vi "Pixmap Probe.vi"(1 "image data":T1) -> (0 "Pause if TRUE":bool)   [LabVIEW 2020]
doc: "Displays the picture and includes information about the width, height, and image color depth of the input picture."
uses:
  <vilib>/picture/picture.llb/imagedata.ctl
panel:
  in  "format string":string="%d bits"
  in  "Tab Control":enum32{"Image   ", "Properties     "}(tab)
  out "Picture":picture
  in  "system palette":string="No color table information included. Default system palette will be used."
  out "Two color table":u32[](array[colorbox])
  out "16.4 million colors":picture
  out "Image Color Depth:":string
  out "256 color table":u32[][](array[colorbox])
  out "Height:":i16
  out "Width:":i16
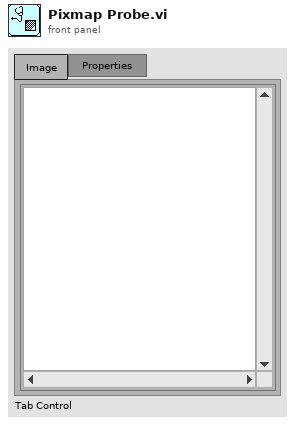
[diagram p1: front panel]
types:
  T1 = typedef "imagedata.ctl" = cluster{"image type":i32, "image depth":i32, "image":u8[], "mask":u8[], "colors":u32[], "Rectangle":cluster{"left":i16, "top":i16, "right":i16, "bottom":i16}}
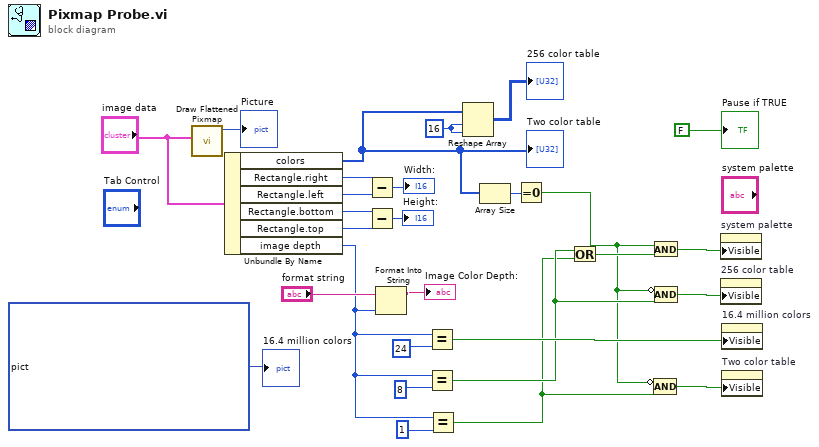
[diagram p0: block diagram]
diagram:
  w3 = 16 ("dimension size")
  n1 = call <vilib>:"Draw Flattened Pixmap.vi"("image data"="image data") -> ("new picture"=→"Picture":picture)  [unwired: 8 in]
  n2 = Unbundle By Name("image data") -> ("colors"=w9:u32[], "Rectangle.right"=w27:i16, "Rectangle.left"=w26:i16, "Rectangle.bottom"=w24:i16, "Rectangle.top"=w23:i16, "image depth"=w10:i32)
  "Two color table" <- w9
  n3 = Subtract(x=w27, y=w26) -> (x-y=→"Width:":i16)
  n4 = Subtract(x=w24, y=w23) -> (x-y=→"Height:":i16)
  n5 = Format Into String(format string="format string", w10) -> (resulting string=→"Image Color Depth:":string)  [unwired: 2 in, 1 out]
  n6 = Equal?(x=w10, y=u8 24) -> (x = y?=w12:bool)
  n7 = Equal?(x=w10, y=u8 8) -> (x = y?=w6:bool)
  n8 = Equal?(x=w10, y=u8 1) -> (x = y?=w1:bool)
  n9 = Reshape Array(w9, w3, w3) -> (→"256 color table":u32[][])
  n10 = Array Size(array=w9) -> (size(s)=w19:i32)
  n11 = Equal To 0?(x=w19) -> (x = 0?=w4:bool)
  n12 = Or(x=w6, y=w1) -> (x .or. y?=w11:bool)
  n13 = And(x=w4, y=w11) -> (x .and. y?=w18:bool)
  n14 = Compound Arithmetic op=AND(invert w4, w1) -> (w5:bool)
  n15 = Compound Arithmetic op=AND(invert w4, w6) -> (w7:bool)
  n16 = property on="system palette" class="Str"("Visible"=w18) -> ()  [unwired: 2 in, 2 out]
  n17 = property on="256 color table" class="Arr (strict)"("Visible"=w7) -> ()  [unwired: 2 in, 2 out]
  n18 = property on="16.4 million colors" class="Pict"("Visible"=w12) -> ()  [unwired: 2 in, 2 out]
  n19 = property on="Two color table" class="Arr (strict)"("Visible"=w5) -> ()  [unwired: 2 in, 2 out]
  "Pause if TRUE" <- FALSE
  "16.4 million colors" <- picture bytes[196638] ("Picture 2")
